vi "_histInit.vi"(11 "RST Dimensions":dbl[][](array[numeric])) -> (3 "YUR: history":dbl[][][](array[numeric]))   [LabVIEW 2021, in "System.lvclass"]
uses:
  System.lvclass
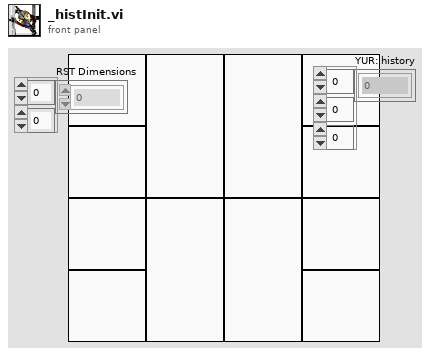
[diagram p1: front panel]
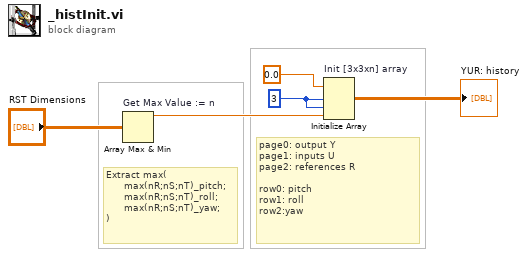
[diagram p0: block diagram]
diagram:
  w1 = 3 ("dimension size")
  # "Extract max(\n      max(nR;nS;nT)_pitch;\n      max(nR;nS;nT)_roll;\n      max(nR;nS;nT)_yaw;\n)"
  # "page0: output Y\npage1: inputs U\npage2: references R\n\nrow0: pitch\nrow1: roll\nrow2:yaw"
  n1 = Array Max & Min "Get Max Value := n"(array="RST Dimensions") -> (max value=w2:dbl)  [unwired: 3 out]
  n2 = Initialize Array "Init [3x3xn] array"(0.0 ("element"), w1, w1, w2) -> (→"YUR: history":dbl[][][])
